vi "Steering_converter.vi"(6 "Yaw":dbl, 9 "setpoint":dbl, 10 "output":dbl, 11 "Degree allowence":dbl) -> (3 "Steer":dbl)   [LabVIEW 2017]
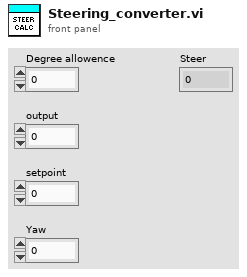
[diagram p1: front panel]
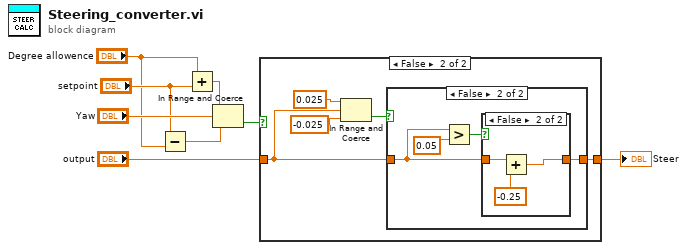
[diagram p0: block diagram]
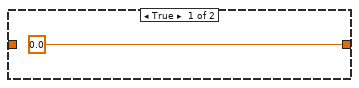
[diagram p2: hidden frame]
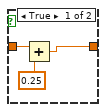
[diagram p4: hidden frame]
diagram:
  n1 = Subtract(x="setpoint", y="Degree allowence") -> (x-y=w2:dbl)
  n2 = Add(x="Degree allowence", y="setpoint") -> (x+y=w4:dbl)
  n3 = In Range and Coerce(upper limit=w4, x="Yaw", lower limit=w2) -> (In Range?=w5:bool)  [unwired: 1 out]
  n4 = case shown="False" w5 {
    tunnel: [0.0 ("t") w11] -> w6
    tunnel: "output" -> [_ w10]
    frame True {
    }
    frame False {
      n5 = In Range and Coerce(upper limit=0.025, x=w10, lower limit=-0.025) -> (In Range?=w14:bool)  [unwired: 1 out]
      n6 = case shown="False" w14 {
        tunnel: [w15 w16] -> w11
        tunnel: w10 -> [w15 w17]
        frame True {
        }
        frame False {
          n7 = Greater?(x=w17, y=0.05) -> (0:w18:bool)
          n8 = case shown="False" w18 {
            tunnel: w17 -> [w21 w24]
            tunnel: [w20 w23] -> w16
            frame True {
              n9 = Add(x=w21, y=0.25) -> (x+y=w20:dbl)
            }
            frame False {
              n10 = Add(x=w24, y=-0.25) -> (x+y=w23:dbl)
            }
          }
        }
      }
    }
  }
  "Steer" <- w6
